vi "onStart.vi"(8 "error in (no error)":errorcluster, 11 "SMO":refnum<class "SMO.lvclass">) -> (0 "error out":errorcluster, 3 "SMO out":refnum<class "SMO.lvclass">)   [LabVIEW 2019, in "SMO.lvclass"]
doc: "JKI State Machine Objects (SMO) 1.3.0.56\nJKI - JKI\nCopyright (c) 2017, JKI"
uses:
  SMO.lvclass
  Dependency/Dependency.lvclass
panel:
  # "For instructions on how to use the JKI State Machine Objects, examples and video tutorials, visit:\nhttp://jki.net/state-machine-objects/\n\nJKI State Machine Objects™\nhttp://jki.net/state-machine-objects/\nCopyright (C) 2005-2015, JKI <info@jki.net>\nALL RIGHTS RESERVED"
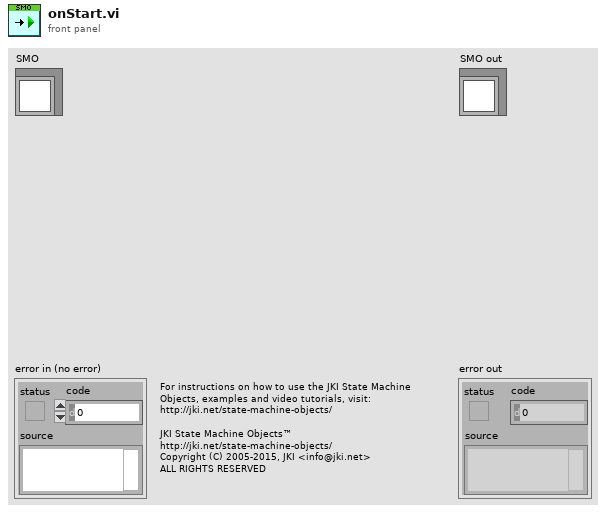
[diagram p1: front panel]
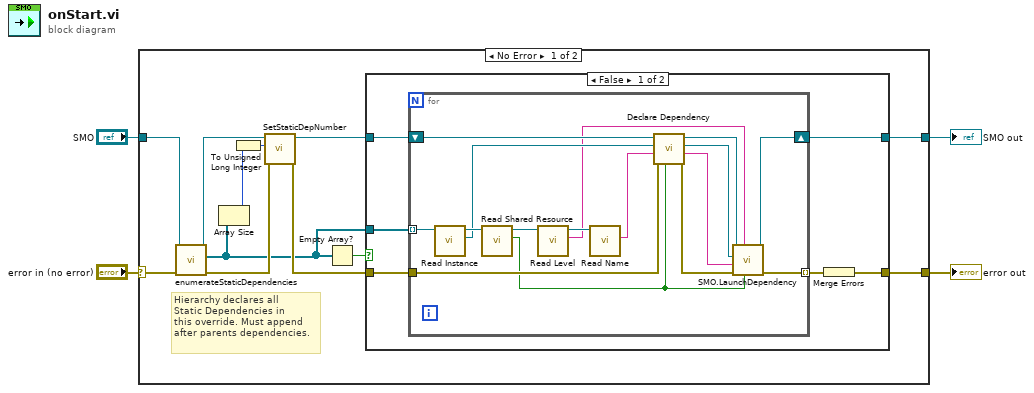
[diagram p0: block diagram]
diagram:
  n1 = case shown="No Error" "error in (no error)" {
    selector: "error in (no error)" -> [w13 w42]
    tunnel: [w15 w42] -> w3
    tunnel: [w16 w41] -> w1
    tunnel: "SMO" -> [w14 w41]
    frame No Error {
      # "Hierarchy declares all\nStatic Dependencies in\nthis override. Must append\nafter parents dependencies."
      n2 = call-dynamic "enumerateStaticDependencies.vi"("error in (no error)"=w13, "SMO"=w14) -> ("error out"=w11:errorcluster, "Static Dependencies"=w5:refnum<class "Dependency.lvclass">[], "SMO out"=w9:refnum<class "SMO.lvclass">)  [unwired: 7 in]
      n3 = Array Size(array=w5) -> (size(s)=w7:i32)
      n4 = To Unsigned Long Integer(number=w7) -> (unsigned 32bit integer=w6:u32)
      n5 = call "SetStaticDepNumber.vi"("error in (no error)"=w11, "Nb of Static Dependencies"=w6, "SMO in"=w9) -> ("error out"=w10:errorcluster, "SMO out"=w8:refnum<class "SMO.lvclass">)  [unwired: 7 in]
      n6 = Empty Array?(array=w5) -> (empty?=w12:bool)
      n7 = case shown="False" w12 {
        tunnel: w5 -> [w22 _]
        tunnel: w8 -> [w17 w40]
        tunnel: w10 -> [w20 w39]
        tunnel: [w19 w40] -> w16
        tunnel: [w18 w39] -> w15
        frame False {
          n8 = for {
            tunnel: w22 -> [w38] mode=indexing
            tunnel: w20 -> [w29]
            tunnel: [w37] -> w21 mode=indexing
            shift-right: [w36] -> w19
            shift-left: w17 -> [w34]
            n9 = call "Read Instance.vi"("Dependency in"=w38) -> ("SMO.lvclass"=w33:refnum<class "SMO.lvclass">, "Dependency out"=w35:refnum<class "Dependency.lvclass">)  [unwired: 9 in]
            n10 = call "Read Shared Resource.vi"("Dependency in"=w35) -> ("Shared Resource"=w28:bool, "Dependency out"=w32:refnum<class "Dependency.lvclass">)  [unwired: 9 in]
            n11 = call "Read Level.vi"("Dependency in"=w32) -> ("Level"=w30:string, "Dependency out"=w31:refnum<class "Dependency.lvclass">)  [unwired: 9 in]
            n12 = call "Read Name.vi"("Dependency in"=w31) -> ("Name"=w27:string)  [unwired: 9 in, 1 out]
            n13 = call "Declare Dependency.vi"("Shared Resource"=w28, "error in (no error)"=w29, "Name"=w27, "Dependency"=w33, "SMO in"=w34) -> ("error out"=w23:errorcluster, "Unique Name"=w24:string, "Dependency out"=w25:refnum<class "SMO.lvclass">, "SMO out"=w26:refnum<class "SMO.lvclass">)  [unwired: 3 in]
            n14 = call "SMO.LaunchDependency.vi"("Shared Resource"=w28, "Level"=w30, "error in (no error)"=w23, "Dependency Name"=w24, "Dependency Type"=w25, "SMO in"=w26) -> ("error out"=w37:errorcluster, "SMO out"=w36:refnum<class "SMO.lvclass">)  [unwired: 2 in, 2 out]
          }
          n15 = Merge Errors(w21) -> (w18:errorcluster)
        }
        frame True {
        }
      }
    }
    frame Error {
    }
  }
  "error out" <- w3
  "SMO out" <- w1
